vi "Simulate Reference Pressures.vi"(8 "error in (no error)":errorcluster, 9 "seconds since 1Jan1904":timestamp, 10 "Pf":dbl, 11 "Pi":dbl) -> (0 "error out":errorcluster, 3 "Simulated Waveform":waveform(dbl))   [LabVIEW 2026, in "Acquisition.lvlib"]
uses:
  Acquisition.lvlib
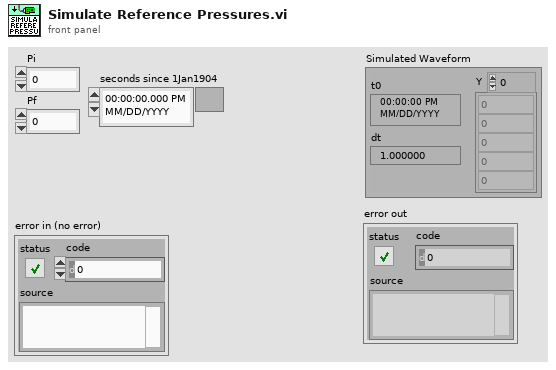
[diagram p1: front panel]
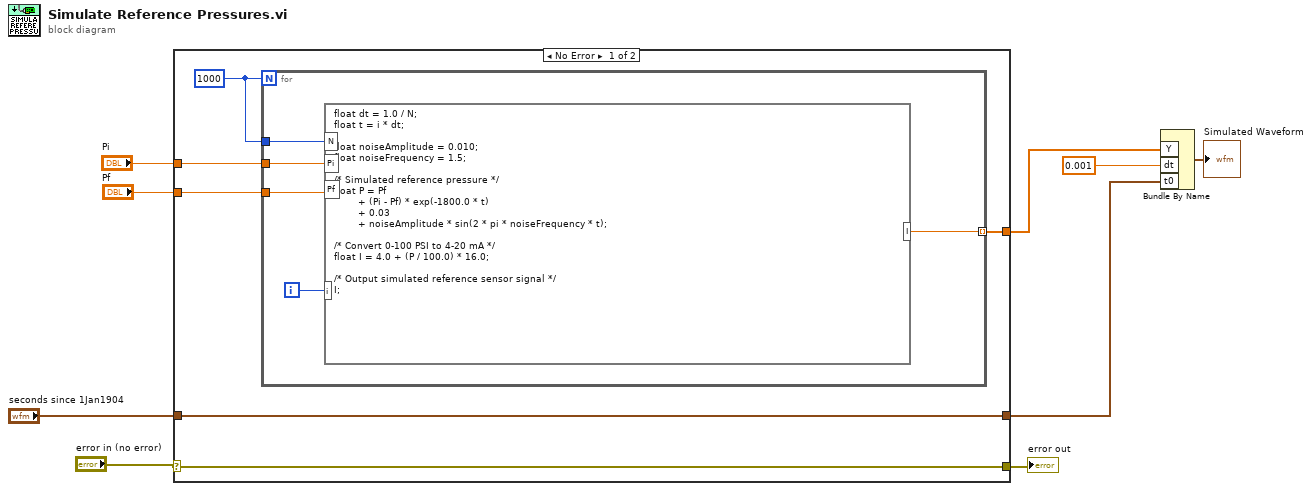
[diagram p0: block diagram]
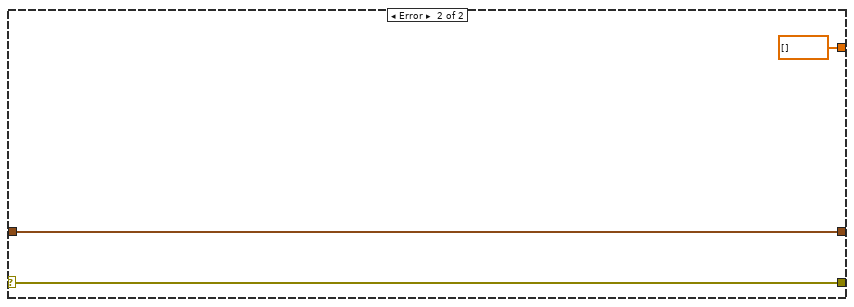
[diagram p2: hidden frame]
diagram:
  n1 = case shown="No Error" "error in (no error)" {
    selector: "error in (no error)" -> [w11 w23]
    tunnel: "Pi" -> [w15 _]
    tunnel: "Pf" -> [w14 _]
    tunnel: [w12 dbl[] []] -> w5
    tunnel: [w11 w23] -> w6
    tunnel: "seconds since 1Jan1904" -> [w10 w21]
    tunnel: [w10 w21] -> w3
    frame No Error {
      w13 = 1000
      n2 = for {
        N: w13 -> [_]
        tunnel: [w19] -> w12 mode=indexing
        tunnel: w15 -> [w18]
        tunnel: w14 -> [w17]
        tunnel: w13 -> [w16]
        i -> [w20]
        n3 = formula code="float dt = 1.0 / N;\nfloat t = i * dt;\n\nfloat noiseAmplitude = 0.010;\nfloat noiseFrequency = 1.5;\n\n/* Simulated reference pressure */\nfloat P = Pf\n        + (Pi - Pf) * exp(-1800.0 * t)\n        + 0.03\n        + noiseAmplitude * sin(2 * pi * noiseFrequency * t);\n\n/* Convert 0-100 PSI to 4-20 mA */\nfloat I = 4.0 + (P / 100.0) * 16.0;\n\n/* Output simulated reference sensor signal */\nI;"("Pi"=w18, "Pf"=w17, "i"=w20, "N"=w16) -> ("I"=w19:dbl)
      }
    }
    frame Error {
    }
  }
  "error out" <- w6
  n4 = Bundle By Name("Y"=w5, "dt"=0.001, "t0"=w3) -> (→"Simulated Waveform":waveform(dbl))  [unwired: 1 in]
